vi "Conditional Error to Warning.vi"(6 "Error Code":i32, 8 "error in":errorcluster) -> (0 "error out":errorcluster)   [LabVIEW 2009, in "POLARIS BME DG.lvlib"]
uses:
  POLARIS BME DG.lvlib
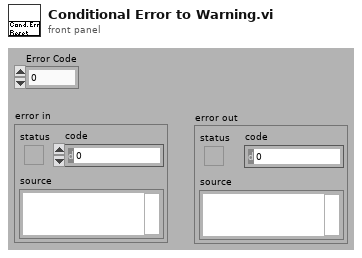
[diagram p1: front panel]
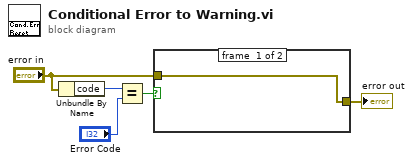
[diagram p0: block diagram]
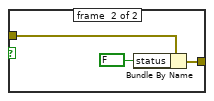
[diagram p2: hidden frame]
diagram:
  n1 = Unbundle By Name("error in") -> ("code"=w2:i32)
  n2 = Equal?(x=w2, y="Error Code") -> (x = y?=w1:bool)
  n3 = case shown="False" w1 {
    tunnel: [w6 w9] -> w5
    tunnel: "error in" -> [w6 w8]
    frame #0 {
    }
    frame #1 {
      n4 = Bundle By Name(cluster=w8, "status"=FALSE) -> (w9:errorcluster)
    }
  }
  "error out" <- w5
